vi "New Component Loader Error.vi"(7 "error source vi name":string, 11 "error":T1) -> (1 "new offset":i32, 3 "error out":errorcluster)   [LabVIEW 2017, in "DSF Core.lvlib" / "Component Loader.lvclass"]
uses:
  Component Loader.lvclass
  Errors.ctl
  <vilib>/NI/Memory Manager/VIs/VIs for Poly/Create Error Cluster (512B).vi
  Shared/Constants/Engine Library Name.vi
  DSF Core.lvlib
  <vilib>/NI/Memory Manager/Deterministic Error Builder.lvlib
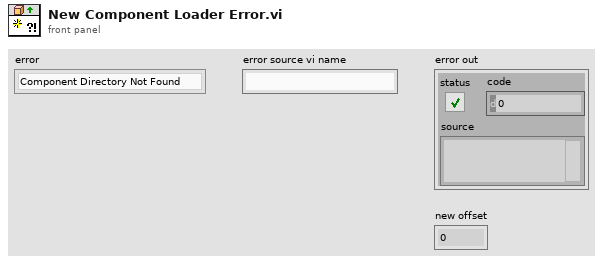
[diagram p1: front panel]
types:
  T1 = typedef "DSF Core.lvlib/Component Loader.lvclass/Errors.ctl" = enum16{"Component Directory Not Found", "Component Not Found", "Class Not Found"}
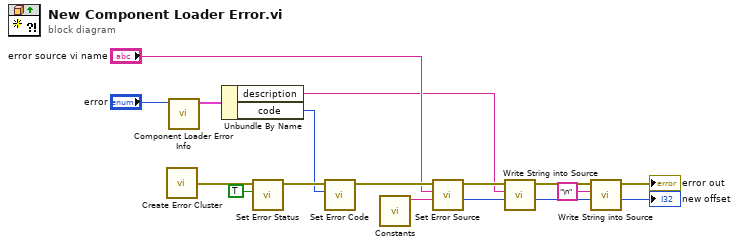
[diagram p0: block diagram]
diagram:
  n1 = call-poly <vilib>:"Create Error Cluster.vi"() -> ("error out"=w16:errorcluster)  [unwired: 1 in]
  n2 = call "Component Loader Error Info.vi"("error"="error") -> ("error info"=w14:cluster{"code":i32, "description":string})  [unwired: 10 in]
  n3 = Unbundle By Name(w14) -> ("description"=w7:string, "code"=w13:i32)
  n4 = call <vilib>:"Set Error Status.vi"("status (T)"=TRUE, "error in"=w16) -> ("error out"=w15:errorcluster)  [unwired: 9 in]
  n5 = call <vilib>:"Set Error Code.vi"("code"=w13, "error in"=w15) -> ("error out"=w12:errorcluster)  [unwired: 9 in]
  n6 = call-poly "Constants.vi"() -> ("Engine Library Name"=w10:string)  [unwired: 11 in]
  n7 = call <vilib>:"Set Error Source.vi"("library name (\"\")"=w10, "vi name"="error source vi name", "error in"=w12) -> ("new offset"=w8:i32, "error out"=w9:errorcluster)  [unwired: 7 in]
  n8 = call <vilib>:"Write String into Source.vi"("offset"=w8, "string"=w7, "error in"=w9) -> ("new offset"=w4:i32, "error out"=w6:errorcluster)  [unwired: 7 in]
  n9 = call <vilib>:"Write String into Source.vi"("offset"=w4, "string"="\n", "error in"=w6) -> ("new offset"=→"new offset":i32, "error out"=→"error out":errorcluster)  [unwired: 7 in]
